vi "LoadConfigData.vi"() -> (3 "Config Data out":T1)   [LabVIEW 2014]
uses:
  <userlib>/_OpenG.lib/array/array.llb/Sort 1D Array (String)__ogtk.vi
  <vilib>/Utility/lvfile.llb/NI_FileType.lvlib
  Config Data.ctl
panel:
  in  "?":string[](array[string])
  in  "Config Typedef in":T1
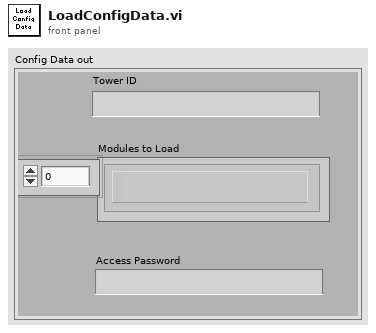
[diagram p1: front panel]
types:
  T1 = typedef "Config Data.ctl" = cluster{"Tower ID":string, "Access Password":string, "Modules to Load":path[]}
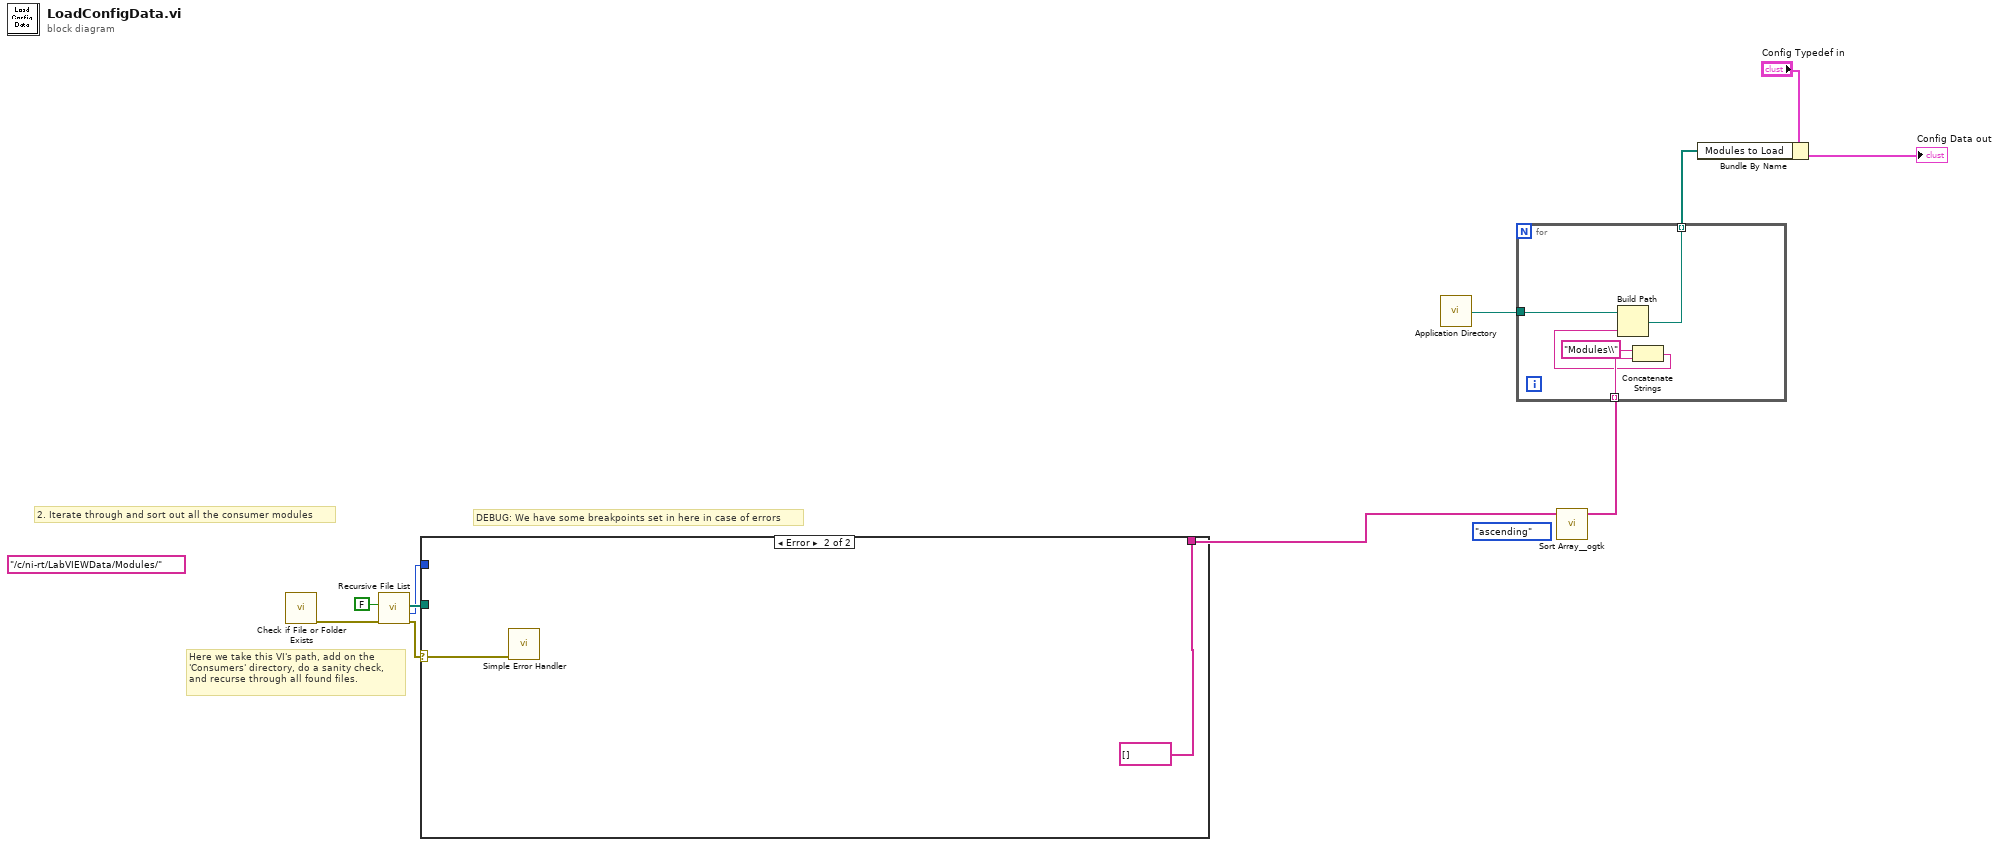
[diagram p0: block diagram]
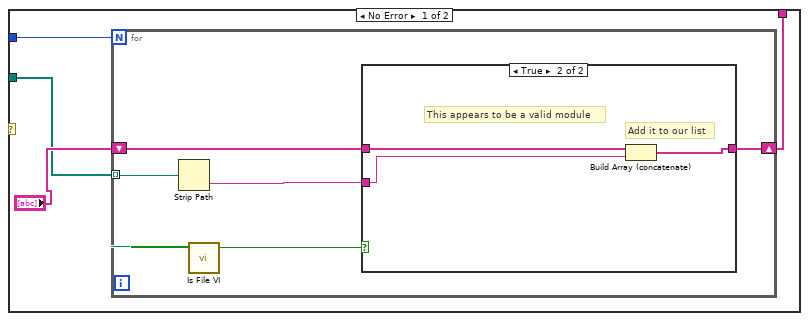
[diagram p2: hidden frame]
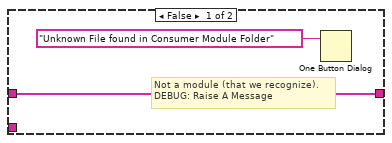
[diagram p3: hidden frame]
diagram:
  w1 = "/c/ni-rt/LabVIEWData/Modules/"
  (unwired) enum16{"ascending", "descending"}."ascending" ("Order")
  # "DEBUG: We have some breakpoints set in here in case of errors"
  # "Here we take this VI's path, add on the\n'Consumers' directory, do a sanity check,\nand recurse through all found files."
  # "2. Iterate through and sort out all the consumer modules"
  n1 = call <vilib>:"Check if File or Folder Exists.vi"() -> ("error out"=w10:errorcluster)  [unwired: 9 in, 2 out]
  n2 = call <vilib>:"Recursive File List.vi"("error in (no error)"=w10, "Treat LLBs as Folders?"=FALSE) -> ("error out"=w7:errorcluster, "Number of Files"=w5:i32, "All Files in Dir"=w8:path[])  [unwired: 5 in, 2 out]
  n3 = case shown="Error" w7 {
    selector: w7 -> [_ w28]
    tunnel: w8 -> [w13 _]
    tunnel: [w16 string[] []] -> w6
    tunnel: w5 -> [w15 _]
    frame No Error {
      n4 = for {
        N: w15 -> [_]
        tunnel: w13 -> [w17] mode=indexing
        shift-right: [w20] -> w16
        shift-left: "?" -> [w19]
        n5 = Strip Path(path=w17) -> (name=w21:string)  [unwired: 1 out]
        n6 = call <vilib>:"Is File VI.vi"("path"=w17) -> ("Is VI?"=w18:bool)  [unwired: 8 in, 2 out]
        n7 = case shown="True" w18 {
          tunnel: w21 -> [_ w24]
          tunnel: [w22 w26] -> w20
          tunnel: w19 -> [w22 w25]
          frame False {
            # "Not a module (that we recognize).\nDEBUG: Raise A Message"
            n8 = One Button Dialog(message="Unknown File found in Consumer Module Folder") -> ()  [unwired: 1 in, 1 out]
          }
          frame True {
            # "Add it to our list"
            # "This appears to be a valid module"
            n9 = Build Array (concatenate)(w25, w24) -> (w26:string[])
          }
        }
      }
    }
    frame Error {
      n10 = call <vilib>:"Simple Error Handler.vi"("error in (no error)"=w28) -> ()  [unwired: 4 in, 5 out]
    }
  }
  n11 = call <vilib>:"Application Directory.vi"() -> ("Application Directory"=w3:path)
  n12 = call-poly <userlib>:"Sort Array__ogtk.vi"("Array in"=w6) -> ("Sorted Array out"=w4:string[])  [unwired: 9 in, 1 out]
  n13 = for {
    tunnel: w4 -> [w31] mode=indexing
    tunnel: w3 -> [w33]
    tunnel: [w32] -> w2 mode=indexing
    n14 = Concatenate Strings("Modules\\" ("string"), w31) -> (w29:string)
    n15 = Build Path(base path=w33, name or relative path=w29) -> (appended path=w32:path)
  }
  n16 = Bundle By Name(cluster="Config Typedef in", "Modules to Load"=w2) -> (→"Config Data out":T1)
